vi "readInLabelsFromXML.vi"(8 "error in (no error)":errorcluster, 10 "NativeXML":refnum<class "NativeXML.lvclass">, 11 "deviceDataBase in":refnum<class "deviceDataBase.lvclass">) -> (0 "error out":errorcluster, 2 "NativeXML out":refnum<class "NativeXML.lvclass">, 3 "deviceDataBase out":refnum<class "deviceDataBase.lvclass">)   [LabVIEW 2011, in "Tools.lvlib" / "DatabaseHelpers.lvlib" / "deviceDataBase.lvclass"]
uses:
  deviceDataBase.lvclass
  NativeXML/NativeXML.lvclass
  deviceDataBase.lvclass/deviceDataBase.ctl
  <vilib>/xml/Close Reference(Node).vi
  <vilib>/xml/NI_XML.lvlib
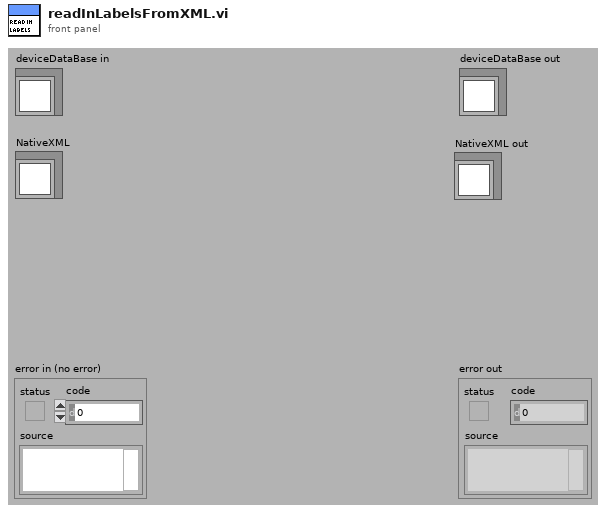
[diagram p1: front panel]
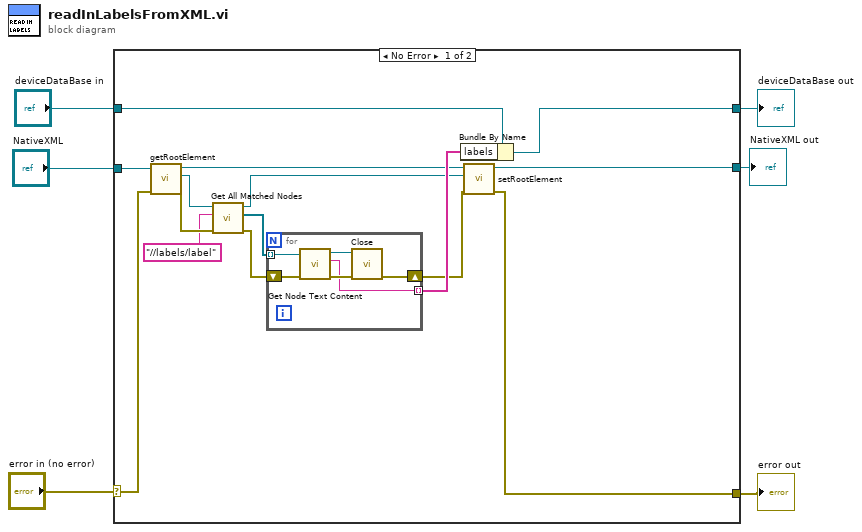
[diagram p0: block diagram]
diagram:
  n1 = case shown="No Error" "error in (no error)" {
    selector: "error in (no error)" -> [w20 w29]
    tunnel: [w8 w29] -> w5
    tunnel: [w12 w28] -> w3
    tunnel: "deviceDataBase in" -> [w13 w28]
    tunnel: "NativeXML" -> [w21 _]
    tunnel: [w7 _] -> w1
    frame No Error {
      n2 = call "getRootElement.vi"("error in (no error)"=w20, "NativeXML in"=w21) -> ("error out"=w19:errorcluster, "RootElement"=w18:refnum<k20>, "NativeXML out"=w11:refnum<class "NativeXML.lvclass">)  [unwired: 7 in]
      n3 = call <vilib>:"Get All Matched Nodes.vi"("error in (no error)"=w19, "XPath expression"="//labels/label", "node in"=w18) -> ("error out"=w15:errorcluster, "node result array"=w16:refnum<k20>[], "node out"=w10:refnum<k20>)  [unwired: 6 in]
      n4 = for {
        tunnel: w16 -> [w27] mode=indexing
        tunnel: [w23] -> w14 mode=indexing
        shift-right: [w22] -> w9
        shift-left: w15 -> [w26]
        n5 = call <vilib>:"Get Node Text Content.vi"("error in (no error)"=w26, "node in"=w27) -> ("error out"=w25:errorcluster, "node text"=w23:string, "node out"=w24:refnum<k20>)  [unwired: 7 in]
        n6 = call-poly <vilib>:"Close.vi"("error in (no error)"=w25, "node"=w24) -> ("error out"=w22:errorcluster)  [unwired: 7 in]
      }
      n7 = Bundle By Name(cluster=w13, "labels"=w14) -> (w12:refnum<class "deviceDataBase.lvclass">)
      n8 = call "setRootElement.vi"("error in (no error)"=w9, "RootElement"=w10, "NativeXML in"=w11) -> ("error out"=w8:errorcluster, "NativeXML out"=w7:refnum<class "NativeXML.lvclass">)  [unwired: 7 in]
    }
    frame Error {
    }
  }
  "error out" <- w5
  "deviceDataBase out" <- w3
  "NativeXML out" <- w1
